vi "initialize debug mode.vi"(10 "User Event in":T1, 11 "editor node in":T2) -> (2 "User Event out":T1, 3 "editor node out":T2, 5 "engine":refnum<data-value>)   [LabVIEW 2013, in "fixed channel tag bus module editor node.lvclass"]
uses:
  fixed channel tag bus module editor node.lvclass
  <vilib>/CEF_TreeControl/Node/NodeRef.ctl
  <vilib>/CEF_TreeControl/Node/NISE_CEF_Node.lvclass
  Configuration Editor/Classes/Engine Parent/Engine Parent Editor Node.lvclass
  <vilib>/CEF_TreeControl/Node/UserEventRef.ctl
  <vilib>/CEF_TreeControl/Controls/EventCluster.ctl
  module/configuration/fixed channel tag bus module configuration.lvclass
  <vilib>/CEF_TreeControl/NISE_CEF_TreeControl.lvlib
  Configuration Editor/Classes/Module editor node/module editor node.lvclass
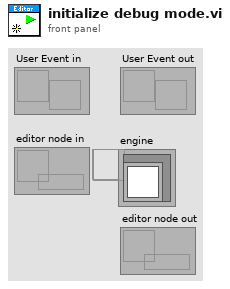
[diagram p1: front panel]
types:
  T1 = typedef "NISE_CEF_Node.lvclass/UserEventRef.ctl" = refnum<user-event>
  T2 = typedef "NISE_CEF_Node.lvclass/NodeRef.ctl" = refnum<data-value>
  T3 = typedef "NISE_CEF_TreeControl.lvlib/EventCluster.ctl" = cluster{"command":string, "data":string}
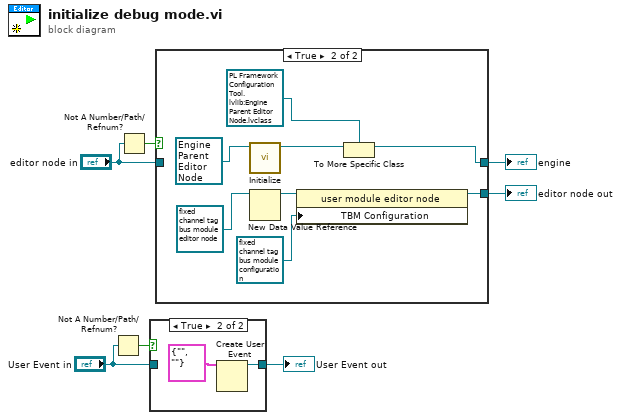
[diagram p0: block diagram]
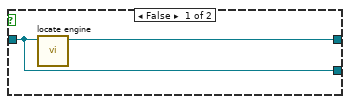
[diagram p3: hidden frame]
diagram:
  n1 = Not A Number/Path/Refnum?(number/path/refnum="User Event in") -> (NaN/Path/Refnum?=w3:bool)
  n2 = Not A Number/Path/Refnum?(number/path/refnum="editor node in") -> (NaN/Path/Refnum?=w4:bool)
  n3 = case shown="True" w3 {
    tunnel: "User Event in" -> [w8 _]
    tunnel: [w8 w9] -> w1
    frame False {
    }
    frame True {
      n4 = Create User Event(user event datatype=T3 {"command"="", "data"=""} ("event data")) -> (user event=w9:refnum<user-event>)  [unwired: 1 in, 1 out]
    }
  }
  "User Event out" <- w1
  n5 = case shown="True" w4 {
    tunnel: "editor node in" -> [w11 _]
    tunnel: [w11 w20] -> w6
    tunnel: [w12 w18] -> w5
    frame False {
      n6 = call "locate engine.vi"("component"=w11) -> ("engine"=w12:refnum<data-value>)  [unwired: 9 in, 1 out]
    }
    frame True {
      n7 = call-dynamic "Initialize.vi"("Engine in"=refnum<class "Engine Parent Editor Node.lvclass"> refnum ("PL Framework Configuration Tool.lvlib:Engine Parent Editor Node.lvclass")) -> ("data value reference"=w19:T2)  [unwired: 8 in, 2 out]
      n8 = New Data Value Reference(data value=refnum<class "fixed channel tag bus module editor node.lvclass"> refnum ("tag bus configurable plugin editor node")) -> (data value reference=w16:refnum<data-value>)  [unwired: 1 in, 1 out]
      n9 = property class="user module editor node"(reference=w16, "TBM Configuration"=refnum<class "fixed channel tag bus module configuration.lvclass"> refnum ("user module configuration")) -> (reference out=w20:refnum<data-value>)  [unwired: 1 in, 1 out]
      n10 = To More Specific Class(target class=refnum<data-value> refnum ("data value reference"), reference=w19) -> (specific class reference=w18:refnum<data-value>)  [unwired: 1 in, 1 out]
    }
  }
  "editor node out" <- w6
  "engine" <- w5
